vi "Get Category.vi"(8 "error in (no error)":errorcluster, 11 "ActiveFrontEndModule editor node in":refnum<class "ActiveFrontEndModule editor node.lvclass">) -> (0 "error out":errorcluster, 2 "Category":string, 3 "ActiveFrontEndModule editor node out":refnum<class "ActiveFrontEndModule editor node.lvclass">)   [LabVIEW 2017, in "ActiveFrontEndModule editor node.lvclass"]
uses:
  ActiveFrontEndModule editor node.lvclass
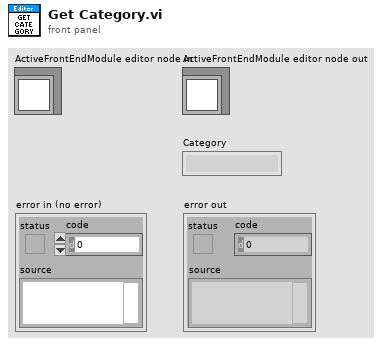
[diagram p1: front panel]
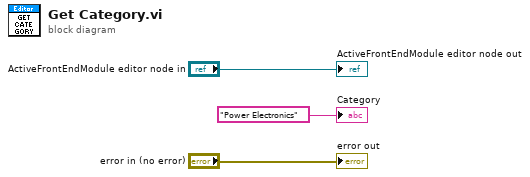
[diagram p0: block diagram]
diagram:
  "error out" <- "error in (no error)"
  "ActiveFrontEndModule editor node out" <- "ActiveFrontEndModule editor node in"
  "Category" <- "Power Electronics" ("Category")
